vi "8Queen_quest.vi"() -> ()   [LabVIEW 2012]
panel:
  out "i":i32
  out "min_past":dbl format="%#_4g"
  out "Solutions":i32
  in  "stop":bool
  in  "soln_dsp":i32
  out "board":bool[][](array[boolean])
  out "loops":i32
  out "all_soln_out":i32[][](array[numeric])
  in  "Q_num":i32=5
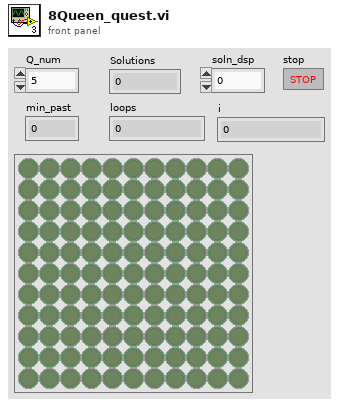
[diagram p1: front panel]
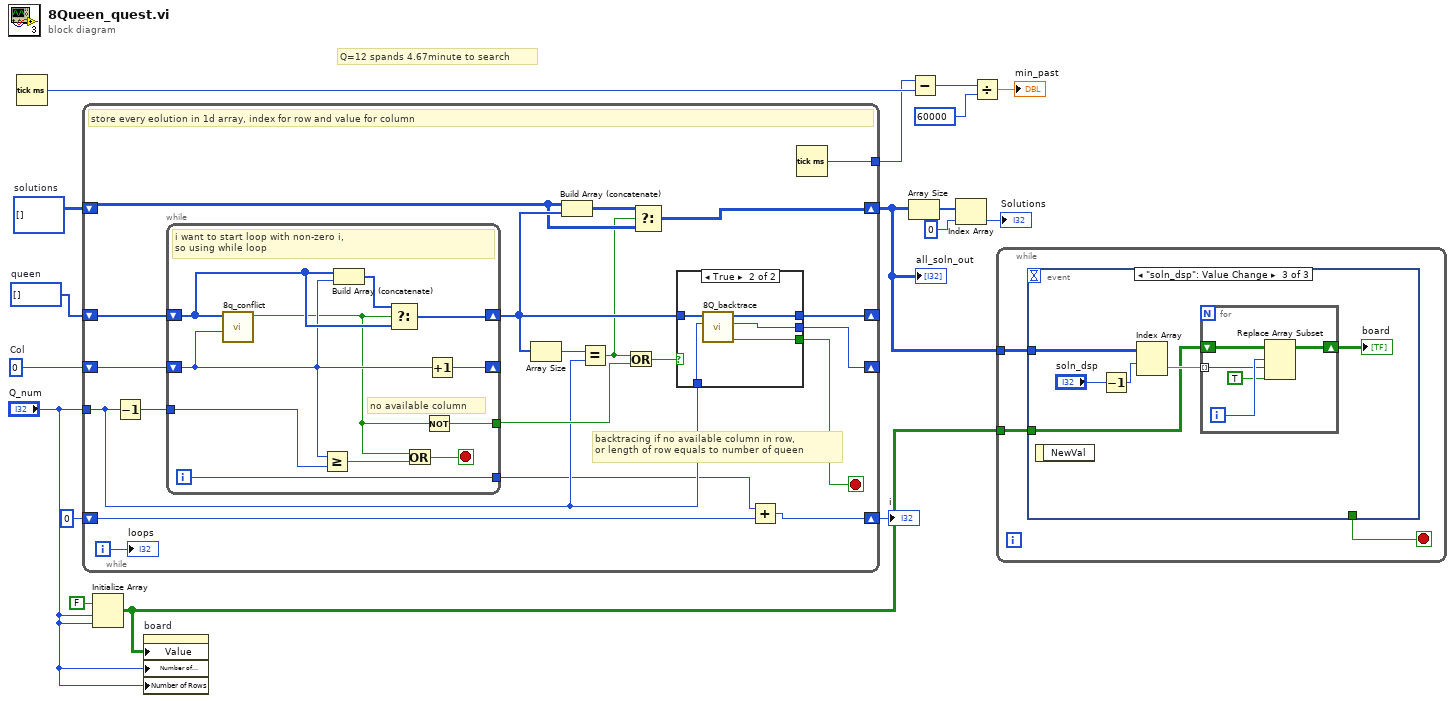
[diagram p0: block diagram]
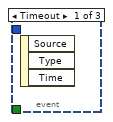
[diagram p2: hidden frame]
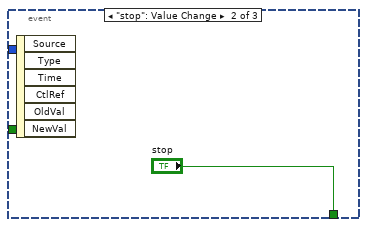
[diagram p3: hidden frame]
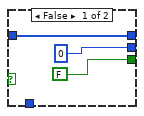
[diagram p4: hidden frame]
diagram:
  w17 = 0  # Col
  w15 = i32[] []  # queen
  w16 = i32[][] []  # solutions
  # "Q=12 spands 4.67minute to search"
  n1 = Tick Count (ms)() -> (millisecond timer value=w4:u32)
  n2 = while {
    shift-right: [w25] -> _
    shift-left: w15 -> [w36]
    shift-right: [w33] -> _
    shift-left: w17 -> [w37]
    tunnel: "Q_num" -> [w22]
    shift-right: [w28] -> w14
    shift-left: w16 -> [w29]
    tunnel: [w21] -> w3
    shift-right: [w19] -> w1
    shift-left: 0 -> [w18]
    i -> [w24]
    stop <- w32 stop-if-true
    # "backtracing if no available column in row,\nor length of row equals to number of queen"
    # "store every eolution in 1d array, index for row and value for column"
    n3 = Decrement(x=w22) -> (x-1=w23:i32)
    n4 = while {
      shift-right: [w54] -> w31
      shift-left: w36 -> [w55]
      shift-right: [w53] -> _
      shift-left: w37 -> [w51]
      tunnel: w23 -> [w52]
      tunnel: [w47] -> w26
      tunnel: [w46] -> w20
      i -> [w46]
      stop <- w49 stop-if-true
      # "no available column"
      # "i want to start loop with non-zero i, \nso using while loop"
      n5 = call "8q_conflict.vi"("nextX"=w51, "State"=w55) -> ("Available"=w48:bool)  [unwired: 9 in]
      n6 = Greater Or Equal?(x=w51, y=w52) -> (x >= y?=w50:bool)
      n7 = Build Array (concatenate)(w55, w51) -> (w56:i32[])
      n8 = Select(t=w56, s=w48, f=w55) -> (s? t:f=w54:i32[])
      n9 = Or(x=w48, y=w50) -> (x .or. y?=w49:bool)
      n10 = Not(x=w48) -> (.not. x?=w47:bool)
      n11 = Increment(x=w51) -> (x+1=w53:i32)
    }
    n12 = Array Size(array=w31) -> (size(s)=w35:i32)
    n13 = Build Array (concatenate)(w29, w31) -> (w30:i32[][])
    n14 = Equal?(x=w35, y=w22) -> (x = y?=w27:bool)
    n15 = Or(x=w27, y=w26) -> (x .or. y?=w34:bool)
    n16 = Select(t=w30, s=w27, f=w29) -> (s? t:f=w28:i32[][])
    n17 = case "backtracing" shown="True" w34 {
      tunnel: [0 ("C") w43] -> w33
      tunnel: w31 -> [w39 w45]
      tunnel: [w39 w44] -> w25
      tunnel: [FALSE ("<0_stop") w42] -> w32
      tunnel: w22 -> [_ w41]
      frame False {
      }
      frame True {
        n18 = call "8Q_backtrace.vi"("Q_Num"=w41, "BT_bfr"=w45) -> ("<0_stop"=w42:bool, "next_start"=w43:i32, "BT_result"=w44:i32[])  [unwired: 7 in]
      }
    }
    n19 = Add(x=w20, y=w18) -> (x+y=w19:i32)
    n20 = Tick Count (ms)() -> (millisecond timer value=w21:u32)
    "loops" <- w24
  }
  "all_soln_out" <- w14
  "i" <- w1
  n21 = Initialize Array(FALSE, "Q_num", "Q_num") -> (w8:bool[][])
  n22 = property on="board" class="Arr (strict)"("Value"=w8, "Number of Columns"="Q_num", "Number of Rows"="Q_num") -> ()  [unwired: 2 in, 2 out]
  n23 = Array Size(array=w14) -> (size(s)=w13:i32[])
  n24 = Subtract(x=w3, y=w4) -> (x-y=w7:u32)
  n25 = Index Array(array=w13, index=0) -> (element=→"Solutions":i32)
  n26 = Divide(x=w7, y=u32 60000) -> (x/y=→"min_past":dbl)
  n27 = while {
    tunnel: w14 -> [w59]
    tunnel: w8 -> [w57]
    stop <- w58 stop-if-true
    n28 = event shown="[2] \"soln_dsp\": Value Change" {
      selector: _ -> [_ _ _]
      dyn-events: _ -> [_ _ _]
      timeout: _ -> [_ _ _]
      tunnel: w59 -> [_ _ w66]
      tunnel: [_ "stop" _] -> w58
      tunnel: w57 -> [_ _ w61]
      event Timeout {
        n29 = event-data() -> ()  [unwired: 1 in, 3 out]
      }
      event "stop": Value Change {
        n30 = event-data() -> ()  [unwired: 1 in, 6 out]
      }
      event "soln_dsp": Value Change {
        n31 = event-data() -> ()  [unwired: 1 in, 1 out]
        n32 = Decrement(x="soln_dsp") -> (x-1=w62:i32)
        n33 = Index Array(array=w66, index (row)=w62) -> (element=w65:i32[])  [unwired: 1 in]
        n34 = for {
          tunnel: w65 -> [w69] mode=indexing
          shift-right: [w68] -> w64
          shift-left: w61 -> [w71]
          i -> [w70]
          n35 = Replace Array Subset(array=w71, new element=TRUE, index (row)=w70, index (col)=w69) -> (w68:bool[][])
        }
        "board" <- w64
      }
    }
  }
